vi "Get BLISS_Update Message Log.vi"(7 "Log History Size (1000)":i32=1000, 8 "error in":errorcluster, 9 "Data Parameters":T1={"Server Index"=0, "username (e.g. name.i@pg.com)"="", "password"="", "Server Status List"=[{"Server Name"="BlissAB101", "data pull successful"=FALSE}], "search criteria"={"views"="", "reject codes"="", "sizes"="", "BLISS Image Types"=enum."Get Both PBQA And Reject Images", "Start Timestamp"=timestamp(0 s since 1904-01-01), "End Timesteamp"=timestamp(0 s since 1904-01-01), "# Images per folder"=1}, "PBQA File List"=[], "Reject File List"=[], "Save to Folder"=path "", "Server List"=[], "Start Time"=timestamp(0 s since 1904-01-01)} {"search criteria"."# Images per folder" min=1 max=10 step=1}, 11 "New Entry":string) -> (0 "error out":errorcluster, 1 "Data Parameters Out":T1={"Server Index"=0, "username (e.g. name.i@pg.com)"="", "password"="", "Server Status List"=[{"Server Name"="BlissAB101", "data pull successful"=FALSE}], "search criteria"={"views"="", "reject codes"="", "sizes"="", "BLISS Image Types"=enum."Get Both PBQA And Reject Images", "Start Timestamp"=timestamp(0 s since 1904-01-01), "End Timesteamp"=timestamp(0 s since 1904-01-01), "# Images per folder"=1}, "PBQA File List"=[], "Reject File List"=[], "Save to Folder"=path "", "Server List"=[], "Start Time"=timestamp(0 s since 1904-01-01)} {"search criteria"."# Images per folder" min=1 max=10 step=1})   [LabVIEW 2018]
uses:
  Get BLISS_Global Variables.vi
  Get BLISS_Data Parameters.ctl
  Get BLISS_Server List 2.ctl
  Get BLISS_Search Criteria.ctl
  Get BLISS_Server Status List.ctl
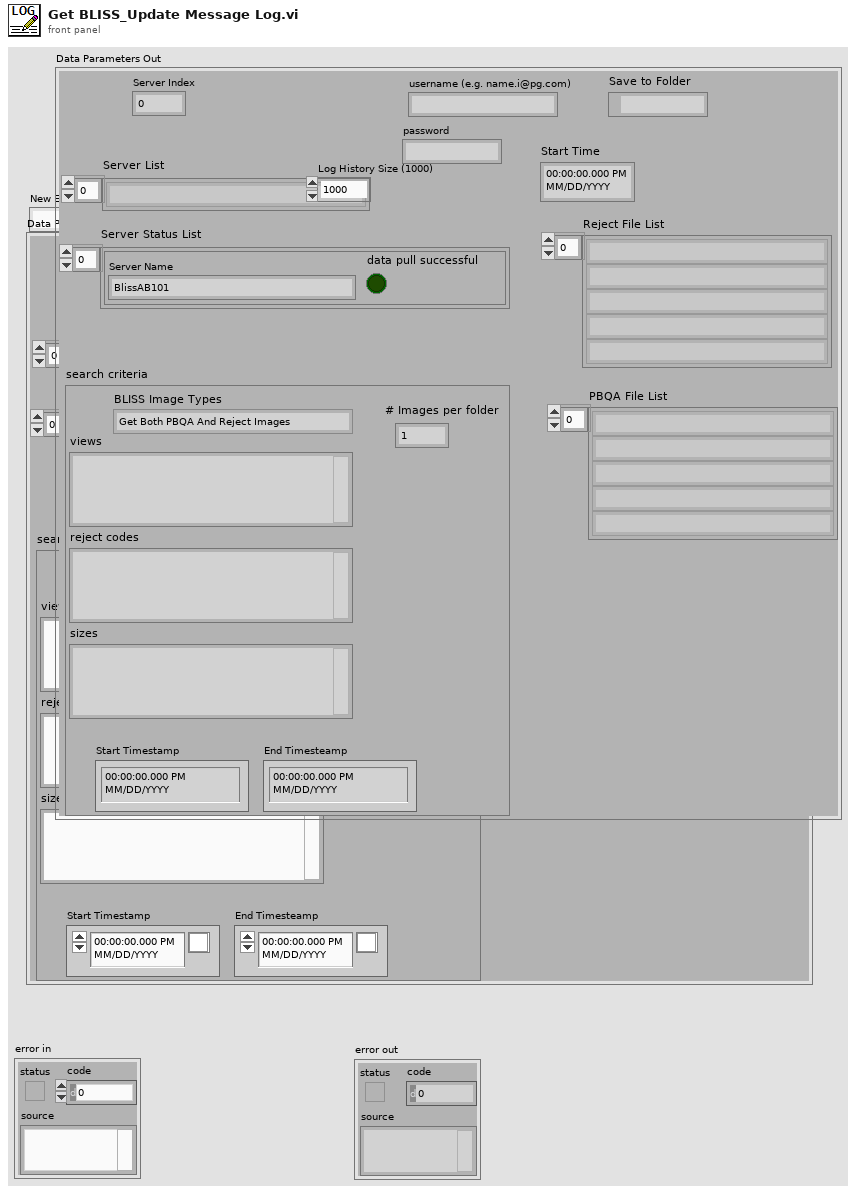
[diagram p1: front panel]
types:
  T1 = typedef "Get BLISS_Data Parameters.ctl" = cluster{"Server Index":i32, "username (e.g. name.i@pg.com)":string, "password":string, "Server Status List":T2, "search criteria":T4, "PBQA File List":string[], "Reject File List":string[], "Save to Folder":path, "Server List":string[], "Start Time":timestamp}
  T2 = typedef "Get BLISS_Server Status List.ctl" = T3[]
  T3 = typedef "Get BLISS_Server List 2.ctl" = cluster{"Server Name":string, "data pull successful":bool}
  T4 = typedef "Get BLISS_Search Criteria.ctl" = cluster{"views":string, "reject codes":string, "sizes":string, "BLISS Image Types":enum16{"Get Only Reject Images", "Get Only PBQA Images", "Get Both PBQA And Reject Images"}, "Start Timestamp":timestamp, "End Timesteamp":timestamp, "# Images per folder":i32}
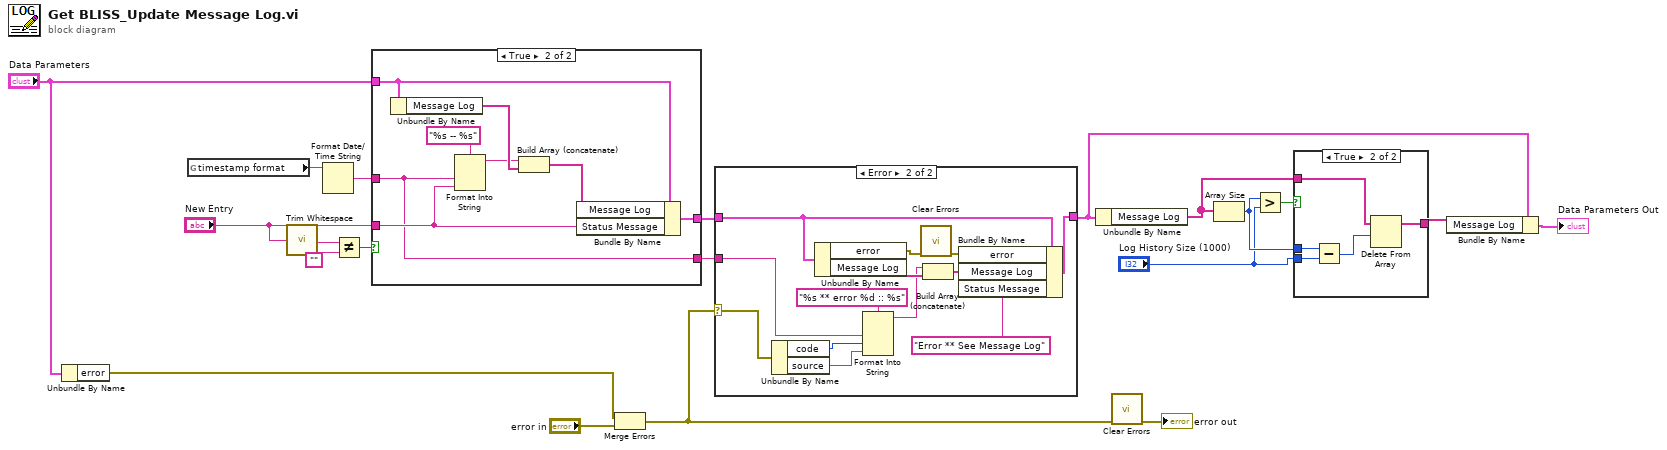
[diagram p0: block diagram]
diagram:
  n1 = Unbundle By Name("Data Parameters") -> ("error"=w16:errorcluster)
  n2 = global read "Get BLISS_Global Variables.vi" "timestamp format"() -> (w1:string)
  n3 = call <vilib>:"Trim Whitespace.vi"("string"="New Entry") -> ("trimmed string"=w17:string)  [unwired: 1 in]
  n4 = Format Date/Time String(time format string (%c)=w1) -> (date/time string=w12:string)  [unwired: 2 in]
  n5 = Not Equal?(x=w17, y="") -> (x != y?=w19:bool)
  n6 = case shown="True" w19 {
    tunnel: [w22 w29] -> w11
    tunnel: "Data Parameters" -> [w22 w26]
    tunnel: w12 -> [w21 w24]
    tunnel: "New Entry" -> [_ w25]
    tunnel: [w21 w24] -> w10
    frame False {
    }
    frame True {
      n7 = Unbundle By Name(w26) -> ("Message Log"=w28:string[])
      n8 = Format Into String(format string="%s -- %s", w24, w25) -> (resulting string=w27:string)  [unwired: 2 in, 1 out]
      n9 = Build Array (concatenate)(w27, w28) -> (w23:string[])
      n10 = Bundle By Name(cluster=w26, "Message Log"=w23, "Status Message"=w25) -> (w29:T1)
    }
  }
  n11 = Merge Errors(w16, "error in") -> (w9:errorcluster)
  n12 = case shown="Error" w9 {
    selector: w9 -> [_ w37]
    tunnel: w11 -> [w31 w43]
    tunnel: [w31 w40] -> w3
    tunnel: w10 -> [_ w34]
    frame No Error {
    }
    frame Error {
      n13 = Unbundle By Name(w37) -> ("code"=w36:i32, "source"=w35:string)
      n14 = Unbundle By Name(w43) -> ("error"=w39:errorcluster, "Message Log"=w42:string[])
      n15 = Format Into String(format string="%s ** error %d :: %s", w34, w36, w35) -> (resulting string=w33:string)  [unwired: 2 in, 1 out]
      n16 = call <vilib>:"Clear Errors.vi"("error in (no error)"=w39) -> ("error out"=w38:errorcluster)  [unwired: 5 in, 1 out]
      n17 = Build Array (concatenate)(w33, w42) -> (w41:string[])
      n18 = Bundle By Name(cluster=w43, "error"=w38, "Message Log"=w41, "Status Message"="Error ** See Message Log") -> (w40:T1)
    }
  }
  n19 = Unbundle By Name(w3) -> ("Message Log"=w6:string[])
  n20 = call <vilib>:"Clear Errors.vi"("error in (no error)"=w9) -> ("error out"=→"error out":errorcluster)  [unwired: 5 in, 1 out]
  n21 = Array Size(array=w6) -> (size(s)=w8:i32)
  n22 = Greater?(x=w8, y="Log History Size (1000)") -> (0:w7:bool)
  n23 = case shown="True" w7 {
    tunnel: w8 -> [_ w50]
    tunnel: "Log History Size (1000)" -> [_ w49]
    tunnel: w6 -> [w45 w47]
    tunnel: [w45 w46] -> w4
    frame False {
    }
    frame True {
      n24 = Subtract(x=w50, y=w49) -> (x-y=w48:i32)
      n25 = Delete From Array(array=w47, length=w48) -> (array with subset deleted=w46:string[])  [unwired: 1 in, 1 out]
    }
  }
  n26 = Bundle By Name(cluster=w3, "Message Log"=w4) -> (→"Data Parameters Out":T1)
